vi "Handle Messages.vi"(8 "error in (no error)":errorcluster, 9 "Message Data":variant, 10 "Message":string, 11 "View In":refnum<class "View.lvclass">) -> (0 "error out":errorcluster, 3 "View Out":refnum<class "View.lvclass">)   [LabVIEW 2020, in "View.lvclass"]
doc: "This is the main method handling incomming messages to the process. This method should be overridden to add functionality to the process or override functionality implemented by a parent. Any message not handled should be sent to the parent method using the default case. \nEach state should be atomic and states should not enqueue new messages from within this method. For cyclic iteration of an action, using a Helper Loop is recommended."
uses:
  View.lvclass
  C:/git/astemes-triarc-framework/source/Framework/Process/Process.lvclass
  Process/Process.lvclass/Process.ctl
  Process/Private/SubVIs/Handle Debug Data.vi
  Logging/Log Debug.vi
  <vilib>/AdvancedString/1D String Array to Delimited String.vi
  <vilib>/Utility/High Resolution Relative Seconds.vi
  Process/Process.lvclass
  C:/git/astemes-triarc-framework/source/Framework/Logging/Logging.lvclass
  Process/Public/Read Name.vi
  <vilib>/Utility/error.llb/Error Cluster From Error Code.vi
  Process/Public/Lifecycle/Get Lifecycle State.vi
  Callback/Callback.lvclass
  Logging/Logging.lvclass
  View.lvclass/View.ctl
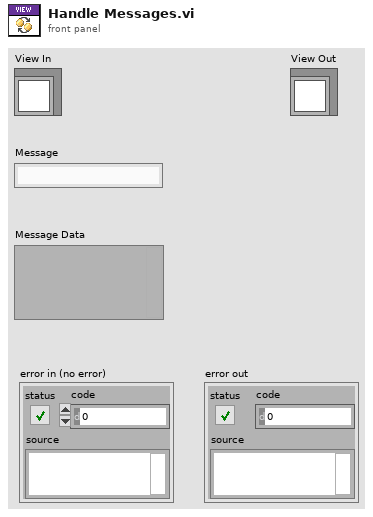
[diagram p1: front panel]
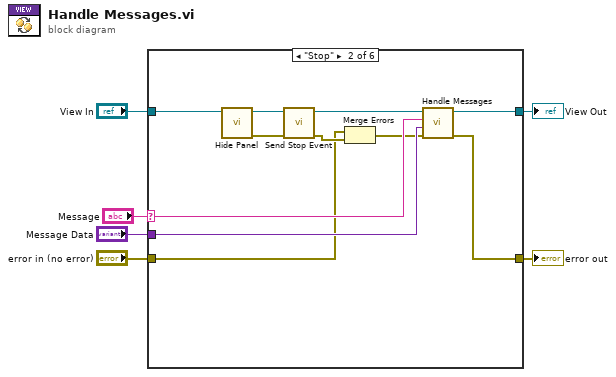
[diagram p0: block diagram]
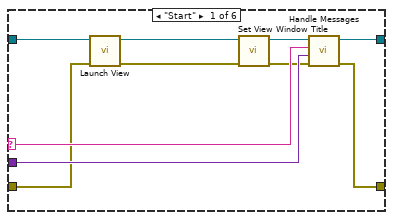
[diagram p2: hidden frame]
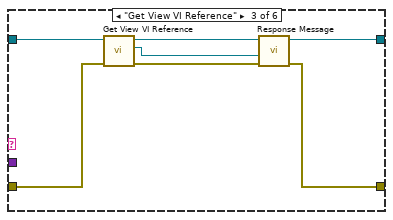
[diagram p3: hidden frame]
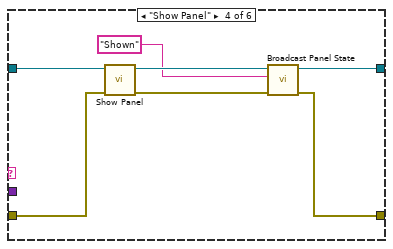
[diagram p4: hidden frame]
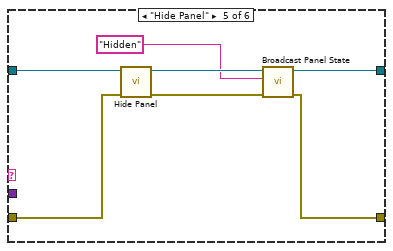
[diagram p5: hidden frame]
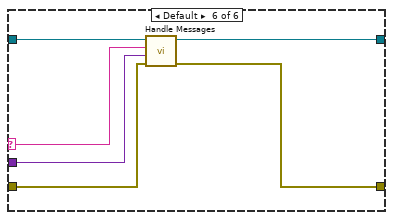
[diagram p6: hidden frame]
diagram:
  n1 = case shown="\"Stop\"" "Message" {
    selector: "Message" -> [w13 w19 _ _ _ w50]
    tunnel: [w14 w23 w33 w38 w45 w54] -> w6
    tunnel: [w15 w21 w34 w36 w43 w53] -> w5
    tunnel: "error in (no error)" -> [w10 w17 w32 w40 w47 w52]
    tunnel: "Message Data" -> [w12 w20 _ _ _ w51]
    tunnel: "View In" -> [w11 w27 w30 w41 w48 w49]
    frame "Start" {
      n2 = call "Launch View.vi"("error in (no error)"=w10, "View In"=w11) -> ("error out"=w8:errorcluster, "View Out"=w9:refnum<class "View.lvclass">)  [unwired: 7 in, 1 out]
      n3 = call "Set View Window Title.vi"("error in (no error)"=w8, "View In"=w9) -> ("error out"=w7:errorcluster, "View Out"=w16:refnum<class "View.lvclass">)  [unwired: 8 in]
      n4 = call-parent "Handle Messages.vi"("error in (no error)"=w7, "Message Data"=w12, "Message"=w13, "Process In"=w16) -> ("error out"=w14:errorcluster, "Process Out"=w15:refnum<class "View.lvclass">)  [unwired: 6 in]
    }
    frame "Stop" {
      n5 = call "Hide Panel.vi"("View In"=w27) -> ("error out"=w25:errorcluster, "View Out"=w26:refnum<class "View.lvclass">)  [unwired: 9 in]
      n6 = call "Send Stop Event.vi"("error in (no error)"=w25, "View In"=w26) -> ("error out"=w24:errorcluster, "View Out"=w22:refnum<class "View.lvclass">)  [unwired: 8 in]
      n7 = Merge Errors(w17, w24) -> (w18:errorcluster)
      n8 = call-parent "Handle Messages.vi"("error in (no error)"=w18, "Message Data"=w20, "Message"=w19, "Process In"=w22) -> ("error out"=w23:errorcluster, "Process Out"=w21:refnum<class "View.lvclass">)  [unwired: 6 in]
    }
    frame "Get View VI Reference" {
      n9 = call "Get View VI Reference.vi"("error in (no error)"=w32, "View In"=w30) -> ("error out"=w31:errorcluster, "View VI Reference"=w28:refnum<vi>, "View Out"=w29:refnum<class "View.lvclass">)  [unwired: 7 in]
      n10 = call "Response Message.vi"("error in (no error)"=w31, "Response Message Data"=w28, "Process In"=w29) -> ("error out"=w33:errorcluster, "Process Out"=w34:refnum<class "View.lvclass">)  [unwired: 7 in]
    }
    frame "Show Panel" {
      n11 = call "Show Panel.vi"("error in (no error)"=w40, "View In"=w41) -> ("error out"=w39:errorcluster, "View Out"=w37:refnum<class "View.lvclass">)  [unwired: 8 in]
      n12 = call "Broadcast Panel State.vi"("error in (no error)"=w39, "Message"="Shown", "View In"=w37) -> ("error out"=w38:errorcluster, "View Out"=w36:refnum<class "View.lvclass">)  [unwired: 7 in]
    }
    frame "Hide Panel" {
      n13 = call "Hide Panel.vi"("error in (no error)"=w47, "View In"=w48) -> ("error out"=w46:errorcluster, "View Out"=w44:refnum<class "View.lvclass">)  [unwired: 8 in]
      n14 = call "Broadcast Panel State.vi"("error in (no error)"=w46, "Message"="Hidden", "View In"=w44) -> ("error out"=w45:errorcluster, "View Out"=w43:refnum<class "View.lvclass">)  [unwired: 7 in]
    }
    frame Default {
      n15 = call-parent "Handle Messages.vi"("error in (no error)"=w52, "Message Data"=w51, "Message"=w50, "Process In"=w49) -> ("error out"=w54:errorcluster, "Process Out"=w53:refnum<class "View.lvclass">)  [unwired: 6 in]
    }
  }
  "error out" <- w6
  "View Out" <- w5
